vi "parking_ung2_loop.vi"() -> ()   [LabVIEW 2012]
uses:
  G_PATH.vi
panel:
  out "parkingpoint":dbl[][](array[numeric])
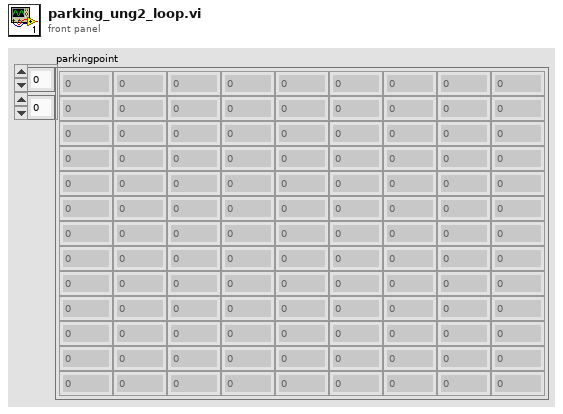
[diagram p1: front panel]
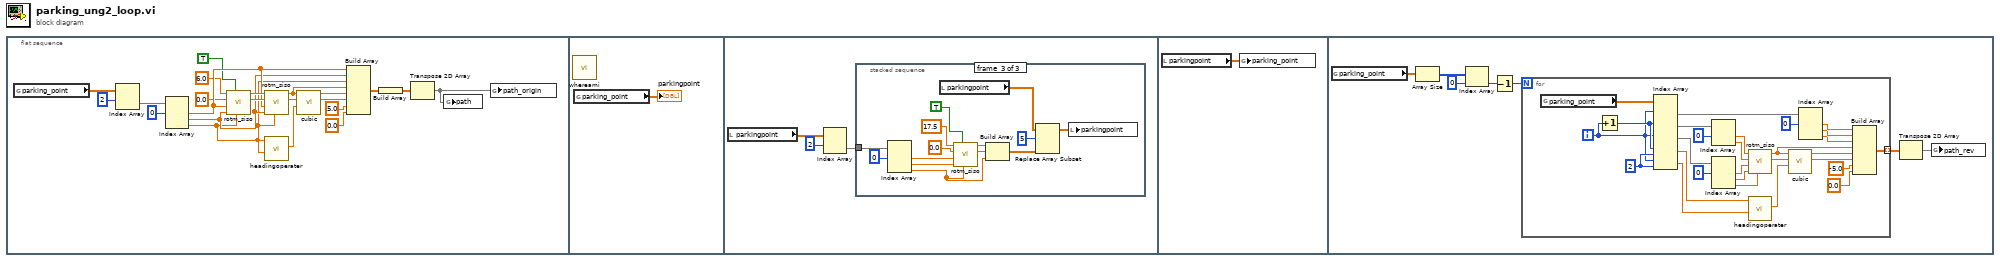
[diagram p0: block diagram]
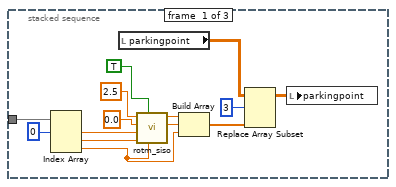
[diagram p2: hidden frame]
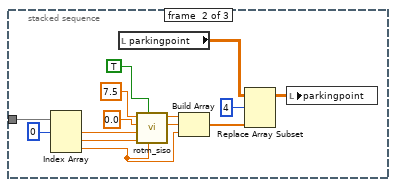
[diagram p3: hidden frame]
diagram:
  n1 = flat-sequence {
    frame #0 {
      n2 = global read "G_PATH.vi" "parking_point"() -> (w1:dbl[][])
      n3 = Index Array(array=w1, index (row)=2) -> (element=w14:dbl[])  [unwired: 1 in]
      n4 = Index Array(array=w14, index #1=0 ("index")) -> (element #1=w18:dbl, element #2=w17:dbl, element #3=w16:dbl)  [unwired: 2 in]
      n5 = call "rotm_siso.vi"("angle[rad]"=w16, "reverse"=TRUE, "y0"=w17, "x0"=w18, "y"=0.0, "x"=6.0) -> ("y'"=w19:dbl, "x'"=w20:dbl)  [unwired: 4 in]
      n6 = call "rotm_siso.vi"("angle[rad]"=w16, "y0"=w17, "x0"=w18, "y"=w19, "x"=w20) -> ("y'"=w9:dbl, "x'"=w3:dbl)  [unwired: 5 in]
      n7 = call "headingoperater.vi"("h1"=w16, "h2"=w16) -> ("h2-h1"=w4:dbl)  [unwired: 8 in, 1 out]
      n8 = call "cubic.vi"("h"=w4, "y"=w9, "x"=w3) -> ("b"=w6:dbl, "a"=w5:dbl)  [unwired: 5 in, 2 out]
      n9 = Build Array(w18, w17, w16, w3, w5, w6, 5.0 ("element"), 0.0 ("element")) -> (w22:dbl[])
      n10 = Build Array(w22) -> (w21:dbl[][])
      n11 = Transpose 2D Array(2D array=w21) -> (transposed array=w2:dbl[][])
      n12 = global write "G_PATH.vi" "path"(w2) -> ()
      n13 = global write "G_PATH.vi" "path_origin"(w2) -> ()
    }
    frame #1 {
      n14 = call "whereami.vi"() -> ()  [unwired: 12 in]
      n15 = global read "G_PATH.vi" "parking_point"() -> (→"parkingpoint":dbl[][])
    }
    frame #2 {
      n16 = local read "parkingpoint"() -> (w24:dbl[][])
      n17 = Index Array(array=w24, index (row)=2) -> (element=w25:dbl[])  [unwired: 1 in]
      n18 = stacked-sequence {
        tunnel: w25 -> [w40 w54 w68]
        frame #0 {
          n19 = Index Array(array=w40, index #1=0 ("index")) -> (element #1=w35:dbl, element #2=w34:dbl, element #3=w29:dbl)  [unwired: 2 in]
          n20 = local read "parkingpoint"() -> (w33:dbl[][])
          n21 = call "rotm_siso.vi"("angle[rad]"=w29, "reverse"=TRUE, "y0"=w34, "x0"=w35, "y"=0.0, "x"=2.5) -> ("y'"=w30:dbl, "x'"=w31:dbl)  [unwired: 4 in]
          n22 = Build Array(w31, w30, w29) -> (w28:dbl[])
          n23 = Replace Array Subset(array=w33, new element=w28, index (row)=3) -> (w27:dbl[][])  [unwired: 1 in]
          n24 = local write "parkingpoint"(w27) -> ()
        }
        frame #1 {
          n25 = Index Array(array=w54, index #1=0 ("index")) -> (element #1=w49:dbl, element #2=w48:dbl, element #3=w43:dbl)  [unwired: 2 in]
          n26 = local read "parkingpoint"() -> (w47:dbl[][])
          n27 = call "rotm_siso.vi"("angle[rad]"=w43, "reverse"=TRUE, "y0"=w48, "x0"=w49, "y"=0.0, "x"=7.5) -> ("y'"=w44:dbl, "x'"=w45:dbl)  [unwired: 4 in]
          n28 = Build Array(w45, w44, w43) -> (w42:dbl[])
          n29 = Replace Array Subset(array=w47, new element=w42, index (row)=4) -> (w41:dbl[][])  [unwired: 1 in]
          n30 = local write "parkingpoint"(w41) -> ()
        }
        frame #2 {
          n31 = Index Array(array=w68, index #1=0 ("index")) -> (element #1=w63:dbl, element #2=w62:dbl, element #3=w57:dbl)  [unwired: 2 in]
          n32 = local read "parkingpoint"() -> (w61:dbl[][])
          n33 = call "rotm_siso.vi"("angle[rad]"=w57, "reverse"=TRUE, "y0"=w62, "x0"=w63, "y"=0.0, "x"=17.5) -> ("y'"=w58:dbl, "x'"=w59:dbl)  [unwired: 4 in]
          n34 = Build Array(w59, w58, w57) -> (w56:dbl[])
          n35 = Replace Array Subset(array=w61, new element=w56, index (row)=5) -> (w55:dbl[][])  [unwired: 1 in]
          n36 = local write "parkingpoint"(w55) -> ()
        }
      }
    }
    frame #3 {
      n37 = local read "parkingpoint"() -> (w69:dbl[][])
      n38 = global write "G_PATH.vi" "parking_point"(w69) -> ()
    }
    frame #4 {
      n39 = global read "G_PATH.vi" "parking_point"() -> (w70:dbl[][])
      n40 = Array Size(array=w70) -> (size(s)=w71:i32[])
      n41 = Index Array(array=w71, index=0) -> (element=w73:i32)
      n42 = Decrement(x=w73) -> (x-1=w74:i32)
      n43 = for {
        N: w74 -> [_]
        tunnel: [w89] -> w75 mode=indexing
        i -> [w97]
        w103 = 2 ("disabled index (col)")
        n44 = global read "G_PATH.vi" "parking_point"() -> (w77:dbl[][])
        n45 = Increment(x=w97) -> (x+1=w104:i32)
        n46 = Index Array(array=w77, index (row) #1=w97, index (row) #2=w104, index (row) #3=w97, index (row) #4=w104, index (col) #4=w103, index (row) #5=w97, index (col) #5=w103) -> (element #1=w96:dbl[], element #2=w87:dbl[], element #3=w83:dbl[], element #4=w102:dbl, element #5=w101:dbl)  [unwired: 3 in]
        n47 = Index Array(array=w87, index #1=0 ("index")) -> (element #1=w86:dbl, element #2=w85:dbl)  [unwired: 1 in]
        n48 = Index Array(array=w83, index #1=0 ("index")) -> (element #1=w82:dbl, element #2=w78:dbl, element #3=w79:dbl)  [unwired: 2 in]
        n49 = call "rotm_siso.vi"("angle[rad]"=w79, "y0"=w78, "x0"=w82, "y"=w85, "x"=w86) -> ("y'"=w80:dbl, "x'"=w81:dbl)  [unwired: 5 in]
        n50 = call "headingoperater.vi"("h1"=w101, "h2"=w102) -> ("h2-h1"=w100:dbl)  [unwired: 8 in, 1 out]
        n51 = call "cubic.vi"("h"=w100, "y"=w80, "x"=w81) -> ("b"=w98:dbl, "a"=w99:dbl)  [unwired: 5 in, 2 out]
        n52 = Index Array(array=w96, index #1=0 ("index")) -> (element #1=w94:dbl, element #2=w93:dbl, element #3=w92:dbl)  [unwired: 2 in]
        n53 = Build Array(w94, w93, w92, w81, w99, w98, -5.0 ("element"), 0.0 ("element")) -> (w89:dbl[])
      }
      n54 = Transpose 2D Array(2D array=w75) -> (transposed array=w76:dbl[][])
      n55 = global write "G_PATH.vi" "path_rev"(w76) -> ()
    }
  }
